vi "svx_Fit Data to Scale.vi"(9 "Cropped Info":cluster{"First Index":i32, "Length":i32}, 10 "Display State In":T1={"X Scale Width %"=50.0, "Y Scale Height %"=50.0, "X-Axis Range"={"Minimum"=0.0, "Maximum"=10.0}, "Y-Axis Range"={"Minimum"=0.0, "Maximum"=10.0}, "Z-Axis Range"={"Minimum"=0.0, "Maximum"=10.0}, "Plot Color"=61212, "Frame Color"=16252785, "Background Color"=16777222, "Initial AutoScale Y"=TRUE, "AutoScale X"=2, "AutoScale Y"=2, "AutoScale Z"=2, "Plot Transparency"=FALSE, "X-Axis Name"="Frequency", "Y-Axis Name"="Amplitude", "Z-Axis Name"="", "X-Axis Scaling Factor"={"Offset"=0.0, "Multiplier"=1.0}, "Y-Axis Scaling Factor"={"Offset"=0.0, "Multiplier"=1.0}, "Z-Axis Scaling Factor"={"Offset"=0.0, "Multiplier"=1.0}, "X-Scale Visible"=TRUE, "Y-Scale Visible"=TRUE, "Z-Scale Visible"=TRUE, "X-Scale Label Visible"=TRUE, "Y-Scale Label Visible"=TRUE, "Z-Scale Label Visible"=TRUE, "X-Axis Range Scaled"={"Minimum"=0.0, "Maximum"=10.0}, "Y-Axis Range Scaled"={"Minimum"=0.0, "Maximum"=10.0}, "Z-Axis Range Scaled"={"Minimum"=0.0, "Maximum"=10.0}, "Rev Z Order"=FALSE, "X-Scale Format Str"="%#.4g", "Y-Scale Format Str"="%#.4g", "Z-Scale Format Str"="%#.4g", "Decor color"=12369084, "Scale Range Change"=refnum, "out of state queue"=refnum, "property nodes"=refnum, "Lines"=[], "Line Properties"={"Line Color"=61212, "Line Width"=61212, "Line Style"=enum."Dash", "DisplayLines"=FALSE}} caption="State" {"Line Properties"."Line Width" min=1}, 11 "Data In":T3={"Dec/Cropped in"={"z0"=0.0, "dz"=1.0, "Plots"=[]}, "Lines"=[]}) -> (0 "Waveform YScale Max":dbl, 1 "Waveform XScale Max":dbl, 2 "Display State Out":T1={"X Scale Width %"=50.0, "Y Scale Height %"=50.0, "X-Axis Range"={"Minimum"=0.0, "Maximum"=10.0}, "Y-Axis Range"={"Minimum"=0.0, "Maximum"=10.0}, "Z-Axis Range"={"Minimum"=0.0, "Maximum"=10.0}, "Plot Color"=61212, "Frame Color"=16252785, "Background Color"=16777222, "Initial AutoScale Y"=TRUE, "AutoScale X"=2, "AutoScale Y"=2, "AutoScale Z"=2, "Plot Transparency"=FALSE, "X-Axis Name"="Frequency", "Y-Axis Name"="Amplitude", "Z-Axis Name"="", "X-Axis Scaling Factor"={"Offset"=0.0, "Multiplier"=1.0}, "Y-Axis Scaling Factor"={"Offset"=0.0, "Multiplier"=1.0}, "Z-Axis Scaling Factor"={"Offset"=0.0, "Multiplier"=1.0}, "X-Scale Visible"=TRUE, "Y-Scale Visible"=TRUE, "Z-Scale Visible"=TRUE, "X-Scale Label Visible"=TRUE, "Y-Scale Label Visible"=TRUE, "Z-Scale Label Visible"=TRUE, "X-Axis Range Scaled"={"Minimum"=0.0, "Maximum"=10.0}, "Y-Axis Range Scaled"={"Minimum"=0.0, "Maximum"=10.0}, "Z-Axis Range Scaled"={"Minimum"=0.0, "Maximum"=10.0}, "Rev Z Order"=FALSE, "X-Scale Format Str"="%#.4g", "Y-Scale Format Str"="%#.4g", "Z-Scale Format Str"="%#.4g", "Decor color"=12369084, "Scale Range Change"=refnum, "out of state queue"=refnum, "property nodes"=refnum, "Lines"=[], "Line Properties"={"Line Color"=61212, "Line Width"=61212, "Line Style"=enum."Dash", "DisplayLines"=FALSE}} caption="State" {"Line Properties"."Line Width" min=1}, 3 "Data Out":T3={"Dec/Cropped in"={"z0"=0.0, "dz"=1.0, "Plots"=[]}, "Lines"=[]}, 4 "Markers":dbl[](array[numeric]), 5 "Y Offset Per spectrum":dbl[](array[numeric]), 7 "Xoffset per spectrum":dbl[](array[numeric]))   [LabVIEW 2017, in "SVX Waterfall Graph.xctl"]
uses:
  <vilib>/addons/_XControls/Waterfall Graph/SVX Waterfall Graph.xctl
  <vilib>/addons/_XControls/Waterfall Graph/subVIs/svx_CroppedData.ctl
  <vilib>/addons/_XControls/Waterfall Graph/subVIs/svx_Waterfall Data.ctl
  <vilib>/addons/_NISVFA/_Shared subVIs/Controls/svc_Cluster of Array of Cluster of XYZ.ctl
  <vilib>/addons/_XControls/Waterfall Graph/subVIs/svx_Waterfall State.ctl
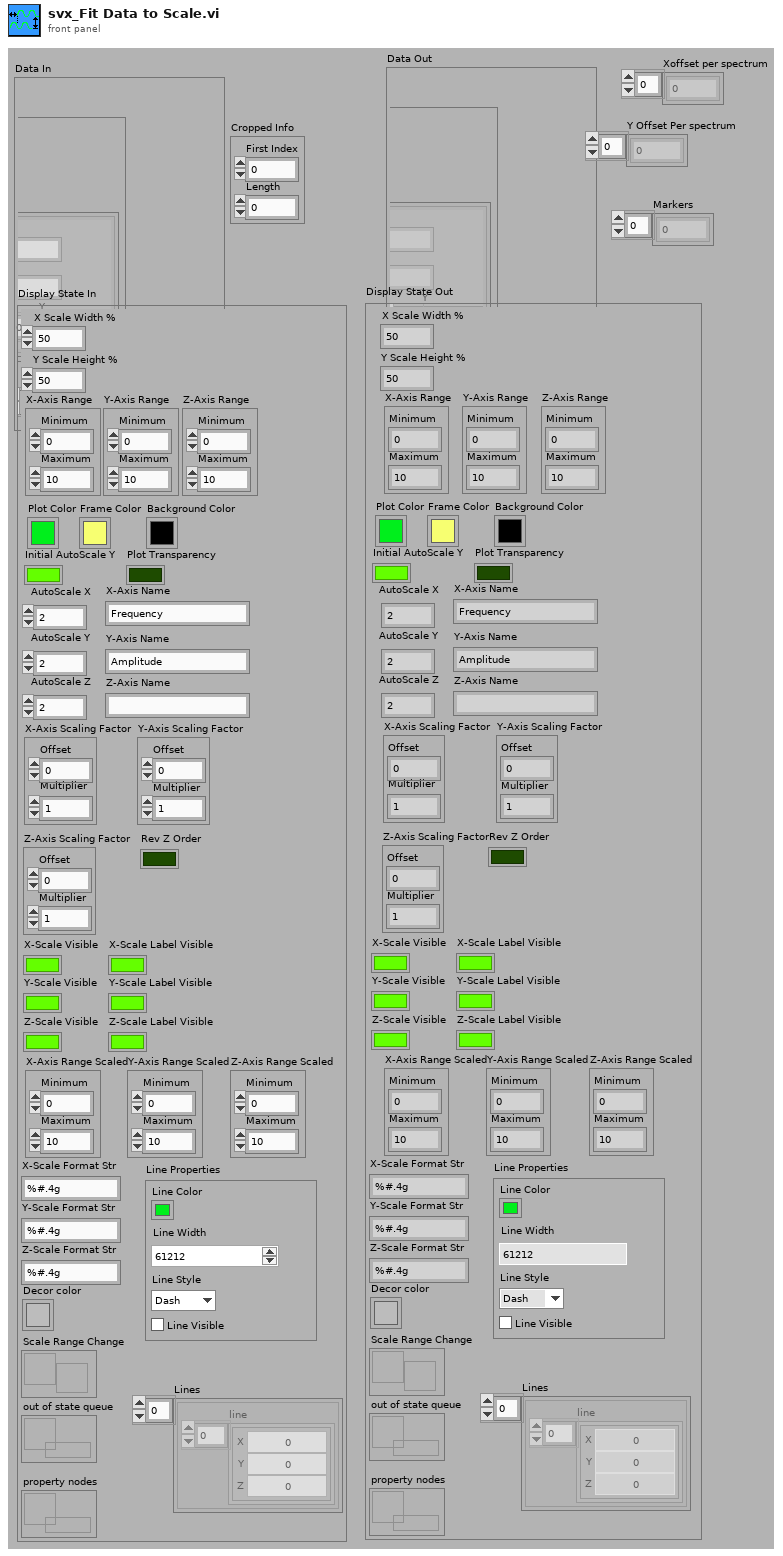
[diagram p1: front panel]
types:
  T1 = typedef "SVX Waterfall Graph.xctl/svx_Waterfall State.ctl" = cluster{"X Scale Width %":dbl, "Y Scale Height %":dbl, "X-Axis Range":cluster{"Minimum":dbl, "Maximum":dbl}, "Y-Axis Range":cluster{"Minimum":dbl, "Maximum":dbl}, "Z-Axis Range":cluster{"Minimum":dbl, "Maximum":dbl}, "Plot Color":u32, "Frame Color":u32, "Background Color":u32, "Initial AutoScale Y":bool, "AutoScale X":u8, "AutoScale Y":u8, "AutoScale Z":u8, "Plot Transparency":bool, "X-Axis Name":string, "Y-Axis Name":string, "Z-Axis Name":string, "X-Axis Scaling Factor":cluster{"Offset":dbl, "Multiplier":dbl}, "Y-Axis Scaling Factor":cluster{"Offset":dbl, "Multiplier":dbl}, "Z-Axis Scaling Factor":cluster{"Offset":dbl, "Multiplier":dbl}, "X-Scale Visible":bool, "Y-Scale Visible":bool, "Z-Scale Visible":bool, "X-Scale Label Visible":bool, "Y-Scale Label Visible":bool, "Z-Scale Label Visible":bool, "X-Axis Range Scaled":cluster{"Minimum":dbl, "Maximum":dbl}, "Y-Axis Range Scaled":cluster{"Minimum":dbl, "Maximum":dbl}, "Z-Axis Range Scaled":cluster{"Minimum":dbl, "Maximum":dbl}, "Rev Z Order":bool, "X-Scale Format Str":string, "Y-Scale Format Str":string, "Z-Scale Format Str":string, "Decor color":u32, "Scale Range Change":refnum<user-event>, "out of state queue":refnum<queue>, "property nodes":refnum<queue>, "Lines":T2[], "Line Properties":cluster{"Line Color":u32, "Line Width":u16, "Line Style":enum32{"Solid", "Dash", "Dot", "DashDot", "DashDotDot"}, "DisplayLines":bool}}
  T2 = typedef "svc_Cluster of Array of Cluster of XYZ.ctl" = cluster{"line":cluster{"X":dbl, "Y":dbl, "Z":dbl}[]}
  T3 = typedef "SVX Waterfall Graph.xctl/svx_CroppedData.ctl" = cluster{"Dec/Cropped in":T4, "Lines":T2[]}
  T4 = typedef "SVX Waterfall Graph.xctl/svx_Waterfall Data.ctl" = cluster{"z0":dbl, "dz":dbl, "Plots":cluster{"x0":dbl, "dx":dbl, "Y":dbl[]}[]}
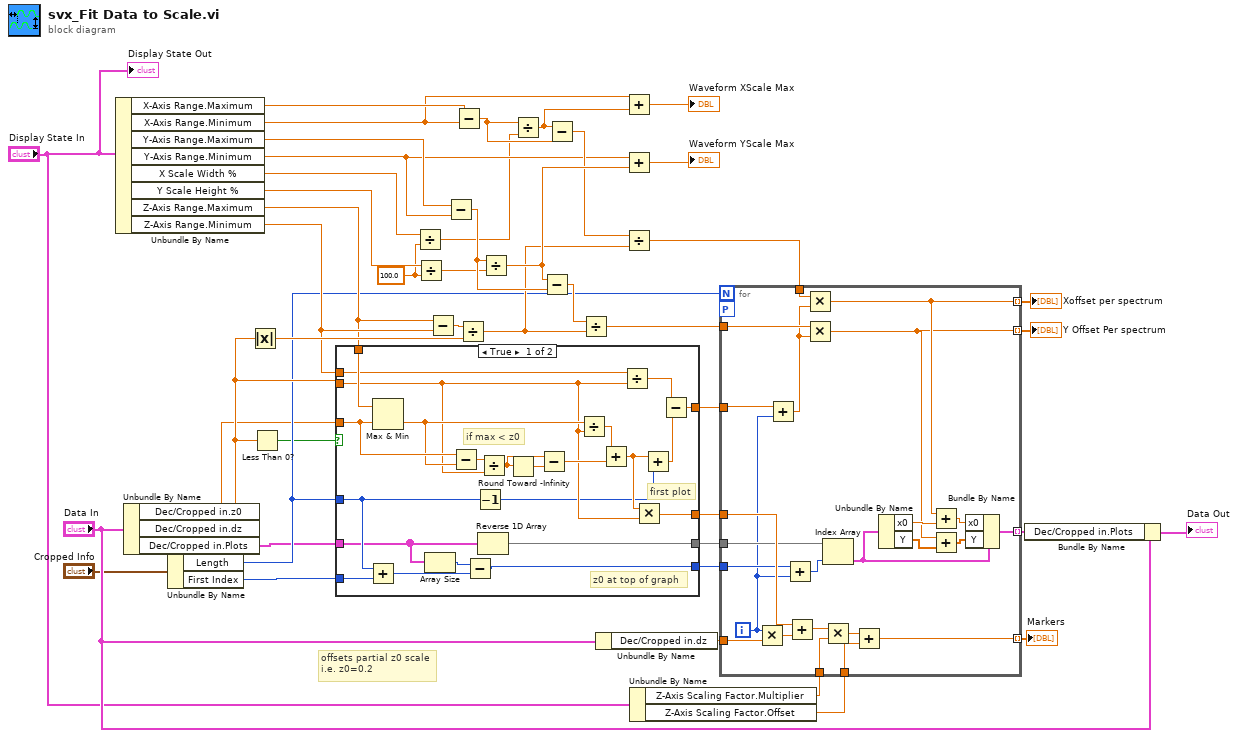
[diagram p0: block diagram]
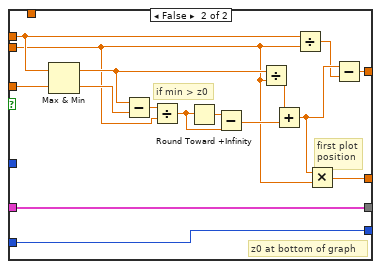
[diagram p2: hidden frame]
diagram:
  w27 = 100.0 ("y")
  # "offsets partial z0 scale\ni.e. z0=0.2"
  n1 = Unbundle By Name("Display State In") -> ("X-Axis Range.Maximum"=w9:dbl, "X-Axis Range.Minimum"=w8:dbl, "Y-Axis Range.Maximum"=w35:dbl, "Y-Axis Range.Minimum"=w34:dbl, "X Scale Width %"=w28:dbl, "Y Scale Height %"=w30:dbl, "Z-Axis Range.Maximum"=w23:dbl, "Z-Axis Range.Minimum"=w24:dbl)
  n2 = Unbundle By Name("Data In") -> ("Dec/Cropped in.z0"=w4:dbl, "Dec/Cropped in.dz"=w22:dbl, "Dec/Cropped in.Plots"=w13:cluster{"x0":dbl, "dx":dbl, "Y":dbl[]}[])
  n3 = Unbundle By Name("Cropped Info") -> ("Length"=w15:i32, "First Index"=w11:i32)
  n4 = Absolute Value(x=w22) -> (abs(x)=w25:dbl)
  n5 = Less Than 0?(x=w22) -> (x < 0?=w14:bool)
  n6 = case shown="True" w14 {
    tunnel: [w67 w83] -> w31
    tunnel: w4 -> [w64 w82]
    tunnel: w24 -> [w63 w81]
    tunnel: w22 -> [w57 w76]
    tunnel: w23 -> [w66 _]
    tunnel: w15 -> [w50 _]
    tunnel: [w59 w77] -> w17
    tunnel: [w52 w70] -> w12
    tunnel: w13 -> [w49 w70]
    tunnel: [w46 w69] -> w10
    tunnel: w11 -> [w51 w69]
    frame True {
      # "if max < z0"
      # "first plot"
      # "z0 at top of graph"
      n7 = Add(x=w50, y=w51) -> (x+y=w47:i32)
      n8 = Max & Min(x=w66, y=w64) -> (min(x,y)=w61:dbl)  [unwired: 1 out]
      n9 = Array Size(array=w49) -> (size(s)=w48:i32)
      n10 = Subtract(x=w64, y=w61) -> (x-y=w55:dbl)
      n11 = Subtract(x=w48, y=w47) -> (x-y=w46:i32)
      n12 = Decrement(x=w50) -> (x-1=w56:i32)
      n13 = Reverse 1D Array(array=w49) -> (reversed array=w52:cluster{"x0":dbl, "dx":dbl, "Y":dbl[]}[])
      n14 = Divide(x=w55, y=w57) -> (x/y=w53:dbl)
      n15 = Round Toward -Infinity(1:w53) -> (0:w54:dbl)
      n16 = Subtract(x=w53, y=w54) -> (x-y=w62:dbl)
      n17 = Divide(x=w61, y=w57) -> (x/y=w60:dbl)
      n18 = Add(x=w60, y=w62) -> (x+y=w58:dbl)
      n19 = Divide(x=w63, y=w57) -> (x/y=w68:dbl)
      n20 = Multiply(x=w58, y=w57) -> (x*y=w59:dbl)
      n21 = Add(x=w58, y=w56) -> (x+y=w65:dbl)
      n22 = Subtract(x=w68, y=w65) -> (x-y=w67:dbl)
    }
    frame False {
      # "if min > z0"
      # "first plot\nposition"
      # "z0 at bottom of graph"
      n23 = Max & Min(x=w81, y=w82) -> (max(x,y)=w79:dbl)  [unwired: 1 out]
      n24 = Subtract(x=w79, y=w82) -> (x-y=w73:dbl)
      n25 = Divide(x=w73, y=w76) -> (x/y=w71:dbl)
      n26 = Round Toward +Infinity(x=w71) -> (ceil(x): smallest int >= x=w72:dbl)
      n27 = Subtract(x=w72, y=w71) -> (x-y=w80:dbl)
      n28 = Divide(x=w79, y=w76) -> (x/y=w78:dbl)
      n29 = Add(x=w78, y=w80) -> (x+y=w75:dbl)
      n30 = Divide(x=w81, y=w76) -> (x/y=w74:dbl)
      n31 = Multiply(x=w75, y=w76) -> (x*y=w77:dbl)
      n32 = Subtract(x=w75, y=w74) -> (x-y=w83:dbl)
    }
  }
  n33 = Divide(x=w28, y=w27) -> (x/y=w26:dbl)
  n34 = Divide(x=w30, y=w27) -> (x/y=w29:dbl)
  n35 = Subtract(x=w23, y=w24) -> (x-y=w33:dbl)
  n36 = Subtract(x=w35, y=w34) -> (x-y=w43:dbl)
  n37 = Subtract(x=w9, y=w8) -> (x-y=w41:dbl)
  n38 = Divide(x=w33, y=w25) -> (x/y=w32:dbl)
  n39 = Divide(x=w43, y=w29) -> (x/y=w45:dbl)
  n40 = Divide(x=w41, y=w26) -> (x/y=w40:dbl)
  n41 = Subtract(x=w45, y=w43) -> (x-y=w44:dbl)
  n42 = Subtract(x=w40, y=w41) -> (x-y=w42:dbl)
  n43 = Divide(x=w44, y=w32) -> (x/y=w38:dbl)
  n44 = Unbundle By Name("Data In") -> ("Dec/Cropped in.dz"=w19:dbl)
  n45 = Add(x=w8, y=w40) -> (x+y=→"Waveform XScale Max":dbl)
  n46 = Add(x=w34, y=w45) -> (x+y=→"Waveform YScale Max":dbl)
  n47 = Divide(x=w42, y=w32) -> (x/y=w39:dbl)
  n48 = Unbundle By Name("Display State In") -> ("Z-Axis Scaling Factor.Multiplier"=w5:dbl, "Z-Axis Scaling Factor.Offset"=w6:dbl)
  n49 = for {
    N: w15 -> [_]
    tunnel: w12 -> [w90]
    tunnel: w39 -> [w107]
    tunnel: [w105] -> w1 mode=indexing
    tunnel: w38 -> [w104]
    tunnel: w31 -> [w102]
    tunnel: w19 -> [w98]
    tunnel: [w91] -> w18 mode=indexing
    tunnel: w17 -> [w96]
    tunnel: w6 -> [w92]
    tunnel: w5 -> [w93]
    tunnel: w10 -> [w88]
    workers-P: _ -> [_]
    tunnel: [w85] -> w2 mode=indexing
    tunnel: [w84] -> w3 mode=indexing
    i -> [w86]
    n50 = Multiply(x=w86, y=w98) -> (x*y=w97:dbl)
    n51 = Add(x=w102, y=w86) -> (x+y=w103:dbl)
    n52 = Add(x=w88, y=w86) -> (x+y=w87:i32)
    n53 = Add(x=w96, y=w97) -> (x+y=w94:dbl)
    n54 = Multiply(x=w107, y=w103) -> (x*y=w85:dbl)
    n55 = Multiply(x=w104, y=w103) -> (x*y=w84:dbl)
    n56 = Index Array(array=w90, index=w87) -> (element=w89:cluster{"x0":dbl, "dx":dbl, "Y":dbl[]})
    n57 = Multiply(x=w94, y=w93) -> (x*y=w95:dbl)
    n58 = Add(x=w95, y=w92) -> (x+y=w91:dbl)
    n59 = Unbundle By Name(w89) -> ("x0"=w99:dbl, "Y"=w101:dbl[])
    n60 = Add(x=w85, y=w99) -> (x+y=w106:dbl)
    n61 = Add(x=w84, y=w101) -> (x+y=w100:dbl[])
    n62 = Bundle By Name(cluster=w89, "x0"=w106, "Y"=w100) -> (w105:cluster{"x0":dbl, "dx":dbl, "Y":dbl[]})
  }
  "Markers" <- w18
  "Y Offset Per spectrum" <- w3
  "Xoffset per spectrum" <- w2
  n63 = Bundle By Name(cluster="Data In", "Dec/Cropped in.Plots"=w1) -> (→"Data Out":T3)
  "Display State Out" <- "Display State In"
